vi "AIM 664 test XML LabVIEW Parser.vi"() -> ()   [LabVIEW 2020]
uses:
  Shared/session_rx_monitor.ctl
  Shared/session_tx_generic.ctl
  Engine/Implementation/Monitor Execution Unit/hardware_channels_rx.ctl
  Engine/Implementation/Monitor Execution Unit/channel_settings_rx.ctl
  <instrlib>/AIM GmbH/_AIM 664/_controls/session_monitor_config.ctl
  Engine/Implementation/Monitor Execution Unit/monitor_queue_settings.ctl
  Engine/Implementation/Tx Execution Unit/hardware_channels_tx.ctl
  Engine/Implementation/Tx Execution Unit/channel_settings_tx.ctl
  Shared/RawFrame.ctl
  <instrlib>/AIM GmbH/_AIM 664/_controls/queue_header_generic.ctl
  Engine/Implementation/Monitor Execution Unit/Monitor Execution Unit.lvclass
  <instrlib>/AIM GmbH/_AIM 664/AIM664LV.lvlib
  Import/AIM ARINC 664 Import.lvlib
  Engine/Implementation/Tx Execution Unit/Tx Generic Execution Unit.lvclass
panel:
  out "error out 2":errorcluster caption="error out"
  out "Tx Generic Configuration":T1 {"channel settings"."Frame Array"."Data" format="%.0x"; "channel settings"."Frame Array"."HeaderInfo"."NetSelect" items=["FDX_TX_FRAME_DLY_A"=0, "FDX_TX_FRAME_DLY_B"=1, "FDX_TX_FRAME_BOTH "=3, "FDX_TX_FRAME_ONLY_A"=4, "FDX_TX_FRAME_ONLY_B "=5]; "channel settings"."Frame Array"."HeaderInfo"."FrameStartMode" items=["FDX_TX_FRAME_START_IFG", "FDX_TX_FRAME_START_PGWT", "FDX_TX_FRAME_START_TRG"]; "channel settings"."Frame Array"."HeaderInfo"."PhysErrorInjection" items=["FDX_TX_FRAME_ERR_OFF"=0, "FDX_TX_FRAME_ERR_CRC"=1, "FDX_TX_FRAME_ERR_ALI"=2, "FDX_TX_FRAME_ERR_PRE"=4, "FDX_TX_FRAME_ERR_PHY"=8]; "channel settings"."Frame Array"."HeaderInfo"."SequenceNumberInit" items=["FDX_TX_FRAME_SEQ_INIT_AUTO"=65535]; "channel settings"."Frame Array"."HeaderInfo"."SequenceNumberOffset" items=["FDX_TX_FRAME_SEQ_OFFS_AUTO "=65535]; "channel settings"."Frame Array"."HeaderInfo"."PayloadGenerationMode" items=["FDX_TX_FRAME_PGM_USER"=0, "FDX_TX_FRAME_PGM_IP_PART"=1, "FDX_TX_FRAME_PGM_IP_FULL"=2, "FDX_TX_FRAME_PGM_IP_PART_TT"=10, "FDX_TX_FRAME_PGM_IP_FULL_TT"=20]; "channel settings"."Frame Array"."HeaderInfo"."PayloadBufferMode" items=["FDX_TX_FRAME_PBM_STD", "FDX_TX_FRAME_PBM_MAC", "FDX_TX_FRAME_PBM_UDP"]}
  in  "get  tx gen - xml in":string
  out "error out":errorcluster
  out "Rx Mon Configuration":T5={"channel #"=0, "channel handle"=0, "InstrumentHandle_board"=0, "InstrumentHandle_port"=0, "Queue ID"=0, "channel settings"={"Monitor Settings"={"DefaultCronoMode"=0, "GlbMonBufferSizeIn"=0}, "Rx Board"=0, "Rx Port"=0}, "File Reference"=refnum, "Monitor Log Directory"="", "monitor queue settings"={"TriggerPosition"=0, "CaptureMode"=0, "Strobe"=0, "MaxFileSize MB (1)"=1}, "Name"=""} {"monitor queue settings"."Strobe" items=["FDX_MON_STROBE_DIS", "FDX_MON_STROBE_STOP", "FDX_MON_STROBE_START"]; "monitor queue settings"."CaptureMode" items=["FDX_MON_SINGLE ", "FDX_MON_CONTINUOUS", "FDX_MON_SELECTIVE", "FDX_MON_RECORDING", "FDX_MON_REROS", "FDX_MON_HMU"]; "channel settings"."Monitor Settings"."DefaultCronoMode" items=["FDX_RX_DEFAULT_ENA_CNT", "FDX_RX_DEFAULT_MON_ENA_ALL", "FDX_RX_DEFAULT_MON_ENA_GOOD"]}
  in  "get  mon - xml in":string
  out "set tx gen out":T9={"QueueSizeIn"=0, "Count"=12, "StartMode"=1} {"StartMode" items=["FDX_STOP", "FDX_START", "FDX_START_TRG", "FDX_START_TIME"]}
  out "error out":errorcluster
  in  "set  tx gen - xml in":string
  out "set xml out":T10={"DefaultCronoMode"=1, "GlbMonBufferSizeIn"=0, "CaptureMode"=0, "MaxFileSizeMB"=1, "Strobe"=0, "TriggerPosition"=0} {"Strobe" items=["FDX_MON_STROBE_DIS", "FDX_MON_STROBE_STOP", "FDX_MON_STROBE_START"]; "CaptureMode" items=["FDX_MON_SINGLE ", "FDX_MON_CONTINUOUS", "FDX_MON_SELECTIVE", "FDX_MON_RECORDING", "FDX_MON_REROS", "FDX_MON_HMU"]; "DefaultCronoMode" items=["FDX_RX_DEFAULT_ENA_CNT", "FDX_RX_DEFAULT_MON_ENA_ALL", "FDX_RX_DEFAULT_MON_ENA_GOOD"]}
  out "error out":errorcluster
  in  "set  mon - xml in":string
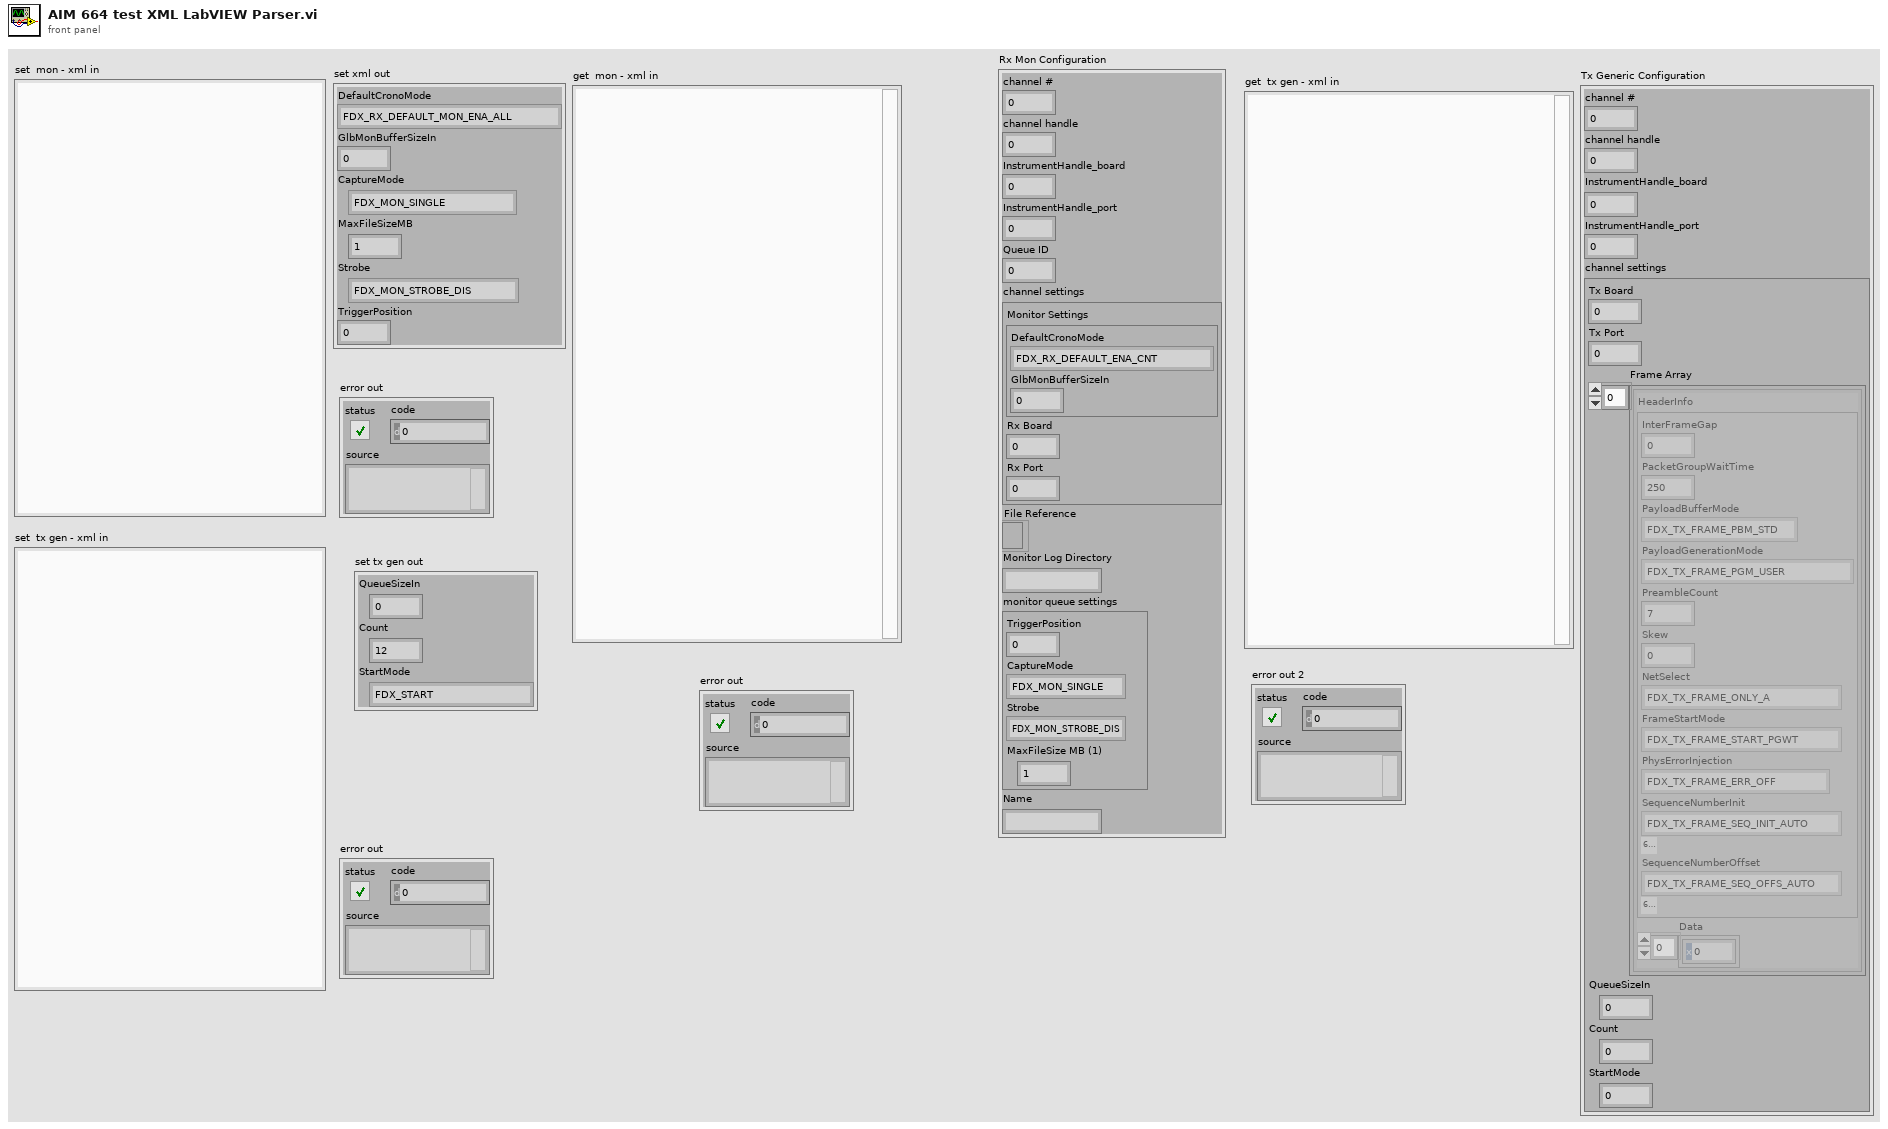
[diagram p1: front panel]
types:
  T1 = typedef "AIM ARINC 664 Engine.lvlib/Implementation.lvlib/Tx Generic Execution Unit.lvclass/hardware_channels_tx.ctl" = cluster{"channel #":u16, "channel handle":u64, "InstrumentHandle_board":u32, "InstrumentHandle_port":u32, "channel settings":T2}
  T2 = typedef "AIM ARINC 664 Engine.lvlib/Implementation.lvlib/Tx Generic Execution Unit.lvclass/channel_settings_tx.ctl" = cluster{"Tx Board":u32, "Tx Port":u32, "Frame Array":T3[], "QueueSizeIn":u32, "Count":u32, "StartMode":u32}
  T3 = typedef "RawFrame.ctl" = cluster{"HeaderInfo":T4, "Data":u8[]}
  T4 = typedef "AIM664LV.lvlib/queue_header_generic.ctl" = cluster{"InterFrameGap":u32, "PacketGroupWaitTime":u32, "PayloadBufferMode":u8, "PayloadGenerationMode":u8, "PreambleCount":u8, "Skew":u32, "NetSelect":u8, "FrameStartMode":u8, "PhysErrorInjection":u32, "SequenceNumberInit":u16, "SequenceNumberOffset":u16}
  T5 = typedef "AIM ARINC 664 Engine.lvlib/Implementation.lvlib/Monitor Execution Unit.lvclass/hardware_channels_rx.ctl" = cluster{"channel #":u16, "channel handle":u64, "InstrumentHandle_board":u32, "InstrumentHandle_port":u32, "Queue ID":u32, "channel settings":T6, "File Reference":refnum<file>, "Monitor Log Directory":string, "monitor queue settings":T8, "Name":string}
  T6 = typedef "AIM ARINC 664 Engine.lvlib/Implementation.lvlib/Monitor Execution Unit.lvclass/channel_settings_rx.ctl" = cluster{"Monitor Settings":T7, "Rx Board":u32, "Rx Port":u32}
  T7 = typedef "AIM664LV.lvlib/session_monitor_config.ctl" = cluster{"DefaultCronoMode":u32, "GlbMonBufferSizeIn":u32}
  T8 = typedef "AIM ARINC 664 Engine.lvlib/Implementation.lvlib/Monitor Execution Unit.lvclass/monitor_queue_settings.ctl" = cluster{"TriggerPosition":u32, "CaptureMode":u32, "Strobe":u32, "MaxFileSize MB (1)":u32}
  T9 = typedef "AIM ARINC 664 Import.lvlib/session_tx_generic.ctl" = cluster{"QueueSizeIn":u32, "Count":i32, "StartMode":i32}
  T10 = typedef "AIM ARINC 664 Import.lvlib/session_rx_monitor.ctl" = cluster{"DefaultCronoMode":u32, "GlbMonBufferSizeIn":u32, "CaptureMode":u32, "MaxFileSizeMB":u32, "Strobe":u32, "TriggerPosition":u32}
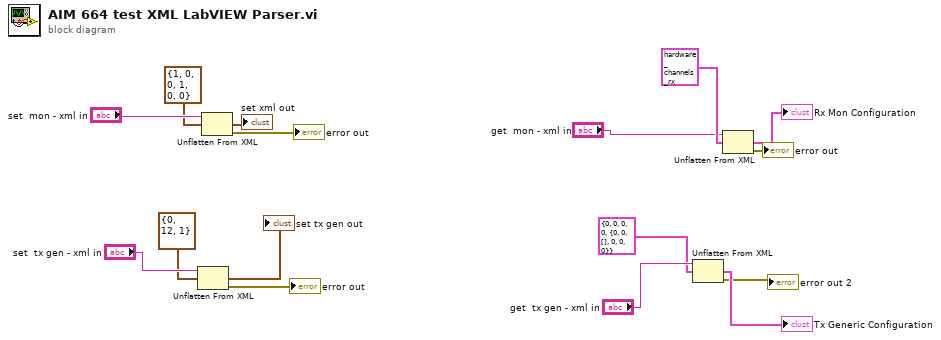
[diagram p0: block diagram]
diagram:
  n1 = Unflatten From XML(xml string="set  tx gen - xml in", type=T9 {"QueueSizeIn"=0, "Count"=12, "StartMode"=1} ("session_tx_generic")) -> (value=→"set tx gen out":T9, error out=→"error out":errorcluster)  [unwired: 1 in]
  n2 = Unflatten From XML(xml string="set  mon - xml in", type=T10 {"DefaultCronoMode"=1, "GlbMonBufferSizeIn"=0, "CaptureMode"=0, "MaxFileSizeMB"=1, "Strobe"=0, "TriggerPosition"=0} ("session_rx_monitor")) -> (value=→"set xml out":T10, error out=→"error out":errorcluster)  [unwired: 1 in]
  n3 = Unflatten From XML(xml string="get  tx gen - xml in", type=T1 {"channel #"=0, "channel handle"=0, "InstrumentHandle_board"=0, "InstrumentHandle_port"=0, "channel settings"={"Tx Board"=0, "Tx Port"=0, "Frame Array"=[], "QueueSizeIn"=0, "Count"=0, "StartMode"=0}} ("Tx cluster out")) -> (value=→"Tx Generic Configuration":T1, error out=→"error out 2":errorcluster)  [unwired: 1 in]
  n4 = Unflatten From XML(xml string="get  mon - xml in", type=T5 {"channel #"=0, "channel handle"=0, "InstrumentHandle_board"=0, "InstrumentHandle_port"=0, "Queue ID"=0, "channel settings"={"Monitor Settings"={"DefaultCronoMode"=1, "GlbMonBufferSizeIn"=0}, "Rx Board"=0, "Rx Port"=1}, "File Reference"=refnum, "Monitor Log Directory"="/home/", "monitor queue settings"={"TriggerPosition"=0, "CaptureMode"=1, "Strobe"=0, "MaxFileSize MB (1)"=1}, "Name"=""} ("RX Parameters")) -> (value=→"Rx Mon Configuration":T5, error out=→"error out":errorcluster)  [unwired: 1 in]
